vi "GeoData.vi"() -> ()   [LabVIEW 2017] (continued)
Currituck\tNC\tCurrituck County\tH1\n27927\t37053\tCorolla\tNC\tCurrituck County\tH1\n27917\t37053\tBarco\tNC\tCurrituck County\tH1\n27941\t37053\tHarbinger\tNC\tCurrituck County\tH1\n27916\t37053\tAydlett\tNC\tCurrituck County\tH1\n27966\t37053\tPowells point\tNC\tCurrituck County\tH1\n27939\t37053\tGrandy\tNC\tCurrituck County\tH1\n27958\t37053\tMoyock\tNC\tCurrituck County\tH1\n27949\t37055\tKitty hawk\tNC\tDare County\tH1\n27968\t37055\tRodanthe\tNC\tDare County\tH1\n27954\t37055\tManteo\tNC\tDare County\tH1\n27953\t37055\tManns harbor\tNC\tDare County\tH1\n27936\t37055\tFrisco\tNC\tDare County\tH1\n27959\t37055\tNags head\tNC\tDare County\tH1\n27981\t37055\tWanchese\tNC\tDare County\tH1\n27948\t37055\tKill devil hills\tNC\tDare County\tH1\n27943\t37055\tHatteras\tNC\tDare County\tH1\n27915\t37055\tAvon\tNC\tDare County\tH1\n27978\t37055\tStumpy point\tNC\tDare County\tH1\n27920\t37055\tBuxton\tNC\tDare County\tH1\n27360\t37057\tThomasville\tNC\tDavidson County\tH1\n27012\t37057\tClemmons\tNC\tDavidson County\tH1\n27374\t37057\tWelcome\tNC\tDavidson County\tH1\n27284\t37057\tKernersville\tNC\tDavidson County\tH1\n27262\t37057\tHigh point\tNC\tDavidson County\tH1\n28127\t37057\tNew london\tNC\tDavidson County\tH1\n27107\t37057\tWinston salem\tNC\tDavidson County\tH1\n27351\t37057\tSouthmont\tNC\tDavidson County\tH1\n27239\t37057\tDenton\tNC\tDavidson County\tH1\n27294\t37057\tLexington\tNC\tDavidson County\tH1\n27373\t37057\tWallburg\tNC\tDavidson County\tH1\n27299\t37057\tLinwood\tNC\tDavidson County\tH1\n27127\t37057\tWinston salem\tNC\tDavidson County\tH1\n27265\t37057\tHigh point\tNC\tDavidson County\tH1\n27292\t37057\tLexington\tNC\tDavidson County\tH1\n27295\t37057\tLexington\tNC\tDavidson County\tH1\n27293\t37057\tLexington\tNC\tDavidson County\tH1\n27014\t37059\tCooleemee\tNC\tDavie County\tH1\n28634\t37059\tHarmony\tNC\tDavie County\tH1\n27028\t37059\tMocksville\tNC\tDavie County\tH1\n27006\t37059\tAdvance\tNC\tDavie County\tH1\n28625\t37059\tStatesville\tNC\tDavie County\tH1\n27055\t37059\tYadkinville\tNC\tDavie County\tH1\n28458\t37061\tRose hill\tNC\tDuplin County\tH1\n28393\t37061\tTurkey\tNC\tDuplin County\tH1\n28365\t37061\tMount olive\tNC\tDuplin County\tH1\n28444\t37061\tHarrells\tNC\tDuplin County\tH1\n28572\t37061\tPink hill\tNC\tDuplin County\tH1\n28325\t37061\tCalypso\tNC\tDuplin County\tH1\n28508\t37061\tAlbertson\tNC\tDuplin County\tH1\n28341\t37061\tFaison\tNC\tDuplin County\tH1\n28453\t37061\tMagnolia\tNC\tDuplin County\tH1\n28525\t37061\tDeep run\tNC\tDuplin County\tH1\n28521\t37061\tChinquapin\tNC\tDuplin County\tH1\n28578\t37061\tSeven springs\tNC\tDuplin County\tH1\n28349\t37061\tKenansville\tNC\tDuplin County\tH1\n28398\t37061\tWarsaw\tNC\tDuplin County\tH1\n28464\t37061\tTeachey\tNC\tDuplin County\tH1\n28574\t37061\tRichlands\tNC\tDuplin County\tH1\n28478\t37061\tWillard\tNC\tDuplin County\tH1\n28518\t37061\tBeulaville\tNC\tDuplin County\tH1\n28466\t37061\tWallace\tNC\tDuplin County\tH1\n27704\t37063\tDurham\tNC\tDurham County\tH1\n27278\t37063\tHillsborough\tNC\tDurham County\tH1\n27503\t37063\tBahama\tNC\tDurham County\tH1\n27701\t37063\tDurham\tNC\tDurham County\tH1\n27709\t37063\tDurham\tNC\tDurham County\tH1\n27717\t37063\tDurham\tNC\tDurham County\tH1\n27712\t37063\tDurham\tNC\tDurham County\tH1\n27707\t37063\tDurham\tNC\tDurham County\tH1\n27713\t37063\tDurham\tNC\tDurham County\tH1\n27706\t37063\tDurham\tNC\tDurham County\tH1\n27560\t37063\tMorrisville\tNC\tDurham County\tH1\n27702\t37063\tDurham\tNC\tDurham County\tH1\n27715\t37063\tDurham\tNC\tDurham County\tH1\n27722\t37063\tDurham\tNC\tDurham County\tH1\n27708\t37063\tDurham\tNC\tDurham County\tH1\n27517\t37063\tChapel hill\tNC\tDurham County\tH1\n27583\t37063\tTimberlake\tNC\tDurham County\tH1\n27613\t37063\tRaleigh\tNC\tDurham County\tH1\n27705\t37063\tDurham\tNC\tDurham County\tH1\n27617\t37063\tRaleigh\tNC\tDurham County\tH1\n27703\t37063\tDurham\tNC\tDurham County\tH1\n27572\t37063\tRougemont\tNC\tDurham County\tH1\n27710\t37063\tDurham\tNC\tDurham County\tH1\n27809\t37065\tBattleboro\tNC\tEdgecombe County\tH1\n27886\t37065\tTarboro\tNC\tEdgecombe County\tH1\n27803\t37065\tRocky mount\tNC\tEdgecombe County\tH1\n27852\t37065\tMacclesfield\tNC\tEdgecombe County\tH1\n27843\t37065\tHobgood\tNC\tEdgecombe County\tH1\n27801\t37065\tRocky mount\tNC\tEdgecombe County\tH1\n27822\t37065\tElm city\tNC\tEdgecombe County\tH1\n27829\t37065\tFountain\tNC\tEdgecombe County\tH1\n27804\t37065\tRocky mount\tNC\tEdgecombe County\tH1\n27891\t37065\tWhitakers\tNC\tEdgecombe County\tH1\n27881\t37065\tSpeed\tNC\tEdgecombe County\tH1\n27819\t37065\tConetoe\tNC\tEdgecombe County\tH1\n27812\t37065\tBethel\tNC\tEdgecombe County\tH1\n27864\t37065\tPinetops\tNC\tEdgecombe County\tH1\n27802\t37065\tRocky mount\tNC\tEdgecombe County\tH1\n27815\t37065\tRocky mount\tNC\tEdgecombe County\tH1\n27834\t37065\tGreenville\tNC\tEdgecombe County\tH1\n27009\t37067\tBelews creek\tNC\tForsyth County\tH1\n27104\t37067\tWinston salem\tNC\tForsyth County\tH1\n27111\t37067\tWinston salem\tNC\tForsyth County\tH1\n27157\t37067\tWinston salem\tNC\tForsyth County\tH1\n27012\t37067\tClemmons\tNC\tForsyth County\tH1\n27021\t37067\tKing\tNC\tForsyth County\tH1\n27043\t37067\tPinnacle\tNC\tForsyth County\tH1\n27106\t37067\tWinston salem\tNC\tForsyth County\tH1\n27199\t37067\tWinston salem\tNC\tForsyth County\tH1\n27045\t37067\tRural hall\tNC\tForsyth County\tH1\n27101\t37067\tWinston salem\tNC\tForsyth County\tH1\n27115\t37067\tWinston salem\tNC\tForsyth County\tH1\n27284\t37067\tKernersville\tNC\tForsyth County\tH1\n27010\t37067\tBethania\tNC\tForsyth County\tH1\n27110\t37067\tWinston salem\tNC\tForsyth County\tH1\n27099\t37067\tRural hall\tNC\tForsyth County\tH1\n27019\t37067\tGermanton\tNC\tForsyth County\tH1\n27052\t37067\tWalnut cove\tNC\tForsyth County\tH1\n27357\t37067\tStokesdale\tNC\tForsyth County\tH1\n27117\t37067\tWinston salem\tNC\tForsyth County\tH1\n27094\t37067\tRural hall\tNC\tForsyth County\tH1\n27150\t37067\tWinston salem\tNC\tForsyth County\tH1\n27108\t37067\tWinston salem\tNC\tForsyth County\tH1\n27107\t37067\tWinston salem\tNC\tForsyth County\tH1\n27235\t37067\tColfax\tNC\tForsyth County\tH1\n27116\t37067\tWinston salem\tNC\tForsyth County\tH1\n27120\t37067\tWinston salem\tNC\tForsyth County\tH1\n27040\t37067\tPfafftown\tNC\tForsyth County\tH1\n27103\t37067\tWinston salem\tNC\tForsyth County\tH1\n27051\t37067\tWalkertown\tNC\tForsyth County\tH1\n27109\t37067\tWinston salem\tNC\tForsyth County\tH1\n27050\t37067\tTobaccoville\tNC\tForsyth County\tH1\n27285\t37067\tKernersville\tNC\tForsyth County\tH1\n27102\t37067\tWinston salem\tNC\tForsyth County\tH1\n27155\t37067\tWinston salem\tNC\tForsyth County\tH1\n27105\t37067\tWinston salem\tNC\tForsyth County\tH1\n27127\t37067\tWinston salem\tNC\tForsyth County\tH1\n27113\t37067\tWinston salem\tNC\tForsyth County\tH1\n27265\t37067\tHigh point\tNC\tForsyth County\tH1\n27023\t37067\tLewisville\tNC\tForsyth County\tH1\n27130\t37067\tWinston salem\tNC\tForsyth County\tH1\n27114\t37067\tWinston salem\tNC\tForsyth County\tH1\n27152\t37067\tWinston salem\tNC\tForsyth County\tH1\n27525\t37069\tFranklinton\tNC\tFranklin County\tH1\n27537\t37069\tHenderson\tNC\tFranklin County\tH1\n27587\t37069\tWake forest\tNC\tFranklin County\tH1\n27508\t37069\tBunn\tNC\tFranklin County\tH1\n27549\t37069\tLouisburg\tNC\tFranklin County\tH1\n27596\t37069\tYoungsville\tNC\tFranklin County\tH1\n27589\t37069\tWarrenton\tNC\tFranklin County\tH1\n27816\t37069\tCastalia\tNC\tFranklin County\tH1\n27544\t37069\tKittrell\tNC\tFranklin County\tH1\n27557\t37069\tMiddlesex\tNC\tFranklin County\tH1\n27597\t37069\tZebulon\tNC\tFranklin County\tH1\n27882\t37069\tSpring hope\tNC\tFranklin County\tH1\n28092\t37071\tLincolnton\tNC\tGaston County\tH1\n28077\t37071\tHigh shoals\tNC\tGaston County\tH1\n28052\t37071\tGastonia\tNC\tGaston County\tH1\n28006\t37071\tAlexis\tNC\tGaston County\tH1\n28101\t37071\tMc adenville\tNC\tGaston County\tH1\n28016\t37071\tBessemer city\tNC\tGaston County\tH1\n28032\t37071\tCramerton\tNC\tGaston County\tH1\n28054\t37071\tGastonia\tNC\tGaston County\tH1\n28080\t37071\tIron station\tNC\tGaston County\tH1\n28098\t37071\tLowell\tNC\tGaston County\tH1\n28034\t37071\tDallas\tNC\tGaston County\tH1\n28055\t37071\tGastonia\tNC\tGaston County\tH1\n28164\t37071\tStanley\tNC\tGaston County\tH1\n28012\t37071\tBelmont\tNC\tGaston County\tH1\n28120\t37071\tMount holly\tNC\tGaston County\tH1\n28021\t37071\tCherryville\tNC\tGaston County\tH1\n28056\t37071\tGastonia\tNC\tGaston County\tH1\n28033\t37071\tCrouse\tNC\tGaston County\tH1\n28053\t37071\tGastonia\tNC\tGaston County\tH1\n28086\t37071\tKings mountain\tNC\tGaston County\tH1\n27938\t37073\tGatesville\tNC\tGates County\tH1\n27969\t37073\tRoduco\tNC\tGates County\tH1\n27946\t37073\tHobbsville\tNC\tGates County\tH1\n27919\t37073\tBelvidere\tNC\tGates County\tH1\n27926\t37073\tCorapeake\tNC\tGates County\tH1\n27937\t37073\tGates\tNC\tGates County\tH1\n27979\t37073\tSunbury\tNC\tGates County\tH1\n27935\t37073\tEure\tNC\tGates County\tH1\n28702\t37075\tAlmond\tNC\tGraham County\tH1\n28733\t37075\tFontana dam\tNC\tGraham County\tH1\n28771\t37075\tRobbinsville\tNC\tGraham County\tH1\n27525\t37077\tFranklinton\tNC\tGranville County\tH1\n27587\t37077\tWake forest\tNC\tGranville County\tH1\n27582\t37077\tStovall\tNC\tGranville County\tH1\n27565\t37077\tOxford\tNC\tGranville County\tH1\n27596\t37077\tYoungsville\tNC\tGranville County\tH1\n27507\t37077\tBullock\tNC\tGranville County\tH1\n27574\t37077\tRoxboro\tNC\tGranville County\tH1\n27522\t37077\tCreedmoor\tNC\tGranville County\tH1\n27581\t37077\tStem\tNC\tGranville County\tH1\n27509\t37077\tButner\tNC\tGranville County\tH1\n27544\t37077\tKittrell\tNC\tGranville County\tH1\n27572\t37077\tRougemont\tNC\tGranville County\tH1\n28530\t37079\tGrifton\tNC\tGreene County\tH1\n28538\t37079\tHookerton\tNC\tGreene County\tH1\n27863\t37079\tPikeville\tNC\tGreene County\tH1\n28501\t37079\tKinston\tNC\tGreene County\tH1\n28554\t37079\tMaury\tNC\tGreene County\tH1\n27888\t37079\tWalstonburg\tNC\tGreene County\tH1\n27828\t37079\tFarmville\tNC\tGreene County\tH1\n27534\t37079\tGoldsboro\tNC\tGreene County\tH1\n28513\t37079\tAyden\tNC\tGreene County\tH1\n27883\t37079\tStantonsburg\tNC\tGreene County\tH1\n28551\t37079\tLa grange\tNC\tGreene County\tH1\n28580\t37079\tSnow hill\tNC\tGreene County\tH1\n27407\t37081\tGreensboro\tNC\tGuilford County\tH1\n27435\t37081\tGreensboro\tNC\tGuilford County\tH1\n27415\t37081\tGreensboro\tNC\tGuilford County\tH1\n27317\t37081\tRandleman\tNC\tGuilford County\tH1\n27310\t37081\tOak ridge\tNC\tGuilford County\tH1\n27403\t37081\tGreensboro\tNC\tGuilford County\tH1\n27408\t37081\tGreensboro\tNC\tGuilford County\tH1\n27455\t37081\tGreensboro\tNC\tGuilford County\tH1\n27425\t37081\tGreensboro\tNC\tGuilford County\tH1\n27417\t37081\tGreensboro\tNC\tGuilford County\tH1\n27268\t37081\tHigh point\tNC\tGuilford County\tH1\n27499\t37081\tGreensboro\tNC\tGuilford County\tH1\n27284\t37081\tKernersville\tNC\tGuilford County\tH1\n27320\t37081\tReidsville\tNC\tGuilford County\tH1\n27262\t37081\tHigh point\tNC\tGuilford County\tH1\n27313\t37081\tPleasant garden\tNC\tGuilford County\tH1\n27357\t37081\tStokesdale\tNC\tGuilford County\tH1\n27358\t37081\tSummerfield\tNC\tGuilford County\tH1\n27377\t37081\tWhitsett\tNC\tGuilford County\tH1\n27410\t37081\tGreensboro\tNC\tGuilford County\tH1\n27420\t37081\tGreensboro\tNC\tGuilford County\tH1\n27413\t37081\tGreensboro\tNC\tGuilford County\tH1\n27214\t37081\tBrowns summit\tNC\tGuilford County\tH1\n27235\t37081\tColfax\tNC\tGuilford County\tH1\n27260\t37081\tHigh point\tNC\tGuilford County\tH1\n27282\t37081\tJamestown\tNC\tGuilford County\tH1\n27261\t37081\tHigh point\tNC\tGuilford County\tH1\n27406\t37081\tGreensboro\tNC\tGuilford County\tH1\n27401\t37081\tGreensboro\tNC\tGuilford County\tH1\n27438\t37081\tGreensboro\tNC\tGuilford County\tH1\n27498\t37081\tGreensboro\tNC\tGuilford County\tH1\n27233\t37081\tClimax\tNC\tGuilford County\tH1\n27263\t37081\tHigh point\tNC\tGuilford County\tH1\n27409\t37081\tGreensboro\tNC\tGuilford County\tH1\n27416\t37081\tGreensboro\tNC\tGuilford County\tH1\n27404\t37081\tGreensboro\tNC\tGuilford County\tH1\n27244\t37081\tElon\tNC\tGuilford County\tH1\n27301\t37081\tMc leansville\tNC\tGuilford County\tH1\n27298\t37081\tLiberty\tNC\tGuilford County\tH1\n27429\t37081\tGreensboro\tNC\tGuilford County\tH1\n27419\t37081\tGreensboro\tNC\tGuilford County\tH1\n27412\t37081\tGreensboro\tNC\tGuilford County\tH1\n27411\t37081\tGreensboro\tNC\tGuilford County\tH1\n27342\t37081\tSedalia\tNC\tGuilford County\tH1\n27497\t37081\tGreensboro\tNC\tGuilford County\tH1\n27215\t37081\tBurlington\tNC\tGuilford County\tH1\n27249\t37081\tGibsonville\tNC\tGuilford County\tH1\n27265\t37081\tHigh point\tNC\tGuilford County\tH1\n27283\t37081\tJulian\tNC\tGuilford County\tH1\n27405\t37081\tGreensboro\tNC\tGuilford County\tH1\n27402\t37081\tGreensboro\tNC\tGuilford County\tH1\n27495\t37081\tGreensboro\tNC\tGuilford County\tH1\n27886\t37083\tTarboro\tNC\tHalifax County\tH1\n27850\t37083\tLittleton\tNC\tHalifax County\tH1\n27843\t37083\tHobgood\tNC\tHalifax County\tH1\n27870\t37083\tRoanoke rapids\tNC\tHalifax County\tH1\n27844\t37083\tHollister\tNC\tHalifax County\tH1\n27890\t37083\tWeldon\tNC\tHalifax County\tH1\n27823\t37083\tEnfield\tNC\tHalifax County\tH1\n27887\t37083\tTillery\tNC\tHalifax County\tH1\n27839\t37083\tHalifax\tNC\tHalifax County\tH1\n27874\t37083\tScotland neck\tNC\tHalifax County\tH1\n27891\t37083\tWhitakers\tNC\tHalifax County\tH1\n28326\t37085\tCameron\tNC\tHarnett County\tH1\n28334\t37085\tDunn\tNC\tHarnett County\tH1\n27330\t37085\tSanford\tNC\tHarnett County\tH1\n27504\t37085\tBenson\tNC\tHarnett County\tH1\n27526\t37085\tFuquay varina\tNC\tHarnett County\tH1\n28368\t37085\tOlivia\tNC\tHarnett County\tH1\n27501\t37085\tAngier\tNC\tHarnett County\tH1\n27592\t37085\tWillow spring\tNC\tHarnett County\tH1\n28323\t37085\tBunnlevel\tNC\tHarnett County\tH1\n27332\t37085\tSanford\tNC\tHarnett County\tH1\n27521\t37085\tCoats\tNC\tHarnett County\tH1\n28356\t37085\tLinden\tNC\tHarnett County\tH1\n28390\t37085\tSpring lake\tNC\tHarnett County\tH1\n27506\t37085\tBuies creek\tNC\tHarnett County\tH1\n27543\t37085\tKipling\tNC\tHarnett County\tH1\n28339\t37085\tErwin\tNC\tHarnett County\tH1\n27505\t37085\tBroadway\tNC\tHarnett County\tH1\n27540\t37085\tHolly springs\tNC\tHarnett County\tH1\n27546\t37085\tLillington\tNC\tHarnett County\tH1\n27552\t37085\tMamers\tNC\tHarnett County\tH1\n28715\t37087\tCandler\tNC\tHaywood County\tH1\n28719\t37087\tCherokee\tNC\tHaywood County\tH1\n28723\t37087\tCullowhee\tNC\tHaywood County\tH1\n28738\t37087\tHazelwood\tNC\tHaywood County\tH1\n28721\t37087\tClyde\tNC\tHaywood County\tH1\n28779\t37087\tSylva\tNC\tHaywood County\tH1\n28785\t37087\tWaynesville\tNC\tHaywood County\tH1\n28745\t37087\tLake junaluska\tNC\tHaywood County\tH1\n28743\t37087\tHot springs\tNC\tHaywood County\tH1\n28716\t37087\tCanton\tNC\tHaywood County\tH1\n28751\t37087\tMaggie valley\tNC\tHaywood County\tH1\n28786\t37087\tWaynesville\tNC\tHaywood County\tH1\n28766\t37089\tPenrose\tNC\tHenderson County\tH1\n28724\t37089\tDana\tNC\tHenderson County\tH1\n28735\t37089\tGerton\tNC\tHenderson County\tH1\n28793\t37089\tHendersonville\tNC\tHenderson County\tH1\n28739\t37089\tHendersonville\tNC\tHenderson County\tH1\n28742\t37089\tHorse shoe\tNC\tHenderson County\tH1\n28784\t37089\tTuxedo\tNC\tHenderson County\tH1\n28758\t37089\tMountain home\tNC\tHenderson County\tH1\n28732\t37089\tFletcher\tNC\tHenderson County\tH1\n28756\t37089\tMill spring\tNC\tHenderson County\tH1\n28731\t37089\tFlat rock\tNC\tHenderson County\tH1\n28790\t37089\tZirconia\tNC\tHenderson County\tH1\n28729\t37089\tEtowah\tNC\tHenderson County\tH1\n28704\t37089\tArden\tNC\tHenderson County\tH1\n28768\t37089\tPisgah forest\tNC\tHenderson County\tH1\n28727\t37089\tEdneyville\tNC\tHenderson County\tH1\n28711\t37089\tBlack mountain\tNC\tHenderson County\tH1\n28710\t37089\tBat cave\tNC\tHenderson County\tH1\n28726\t37089\tEast flat rock\tNC\tHenderson County\tH1\n28760\t37089\tNaples\tNC\tHenderson County\tH1\n28773\t37089\tSaluda\tNC\tHenderson County\tH1\n28791\t37089\tHendersonville\tNC\tHenderson County\tH1\n28759\t37089\tMills river\tNC\tHenderson County\tH1\n28792\t37089\tHendersonville\tNC\tHenderson County\tH1\n27897\t37091\tWoodland\tNC\tHertford County\tH1\n27942\t37091\tHarrellsville\tNC\tHertford County\tH1\n27805\t37091\tAulander\tNC\tHertford County\tH1\n27855\t37091\tMurfreesboro\tNC\tHertford County\tH1\n27910\t37091\tAhoskie\tNC\tHertford County\tH1\n27922\t37091\tCofield\tNC\tHertford County\tH1\n27986\t37091\tWinton\tNC\tHertford County\tH1\n27818\t37091\tComo\tNC\tHertford County\tH1\n28371\t37093\tParkton\tNC\tHoke County\tH1\n28306\t37093\tFayetteville\tNC\tHoke County\tH1\n28315\t37093\tAberdeen\tNC\tHoke County\tH1\n28364\t37093\tMaxton\tNC\tHoke County\tH1\n28304\t37093\tFayetteville\tNC\tHoke County\tH1\n28377\t37093\tRed springs\tNC\tHoke County\tH1\n28386\t37093\tShannon\tNC\tHoke County\tH1\n28376\t37093\tRaeford\tNC\tHoke County\tH1\n28357\t37093\tLumber bridge\tNC\tHoke County\tH1\n27860\t37095\tPantego\tNC\tHyde County\tH1\n27810\t37095\tBelhaven\tNC\tHyde County\tH1\n27875\t37095\tScranton\tNC\tHyde County\tH1\n27826\t37095\tFairfield\tNC\tHyde County\tH1\n27824\t37095\tEngelhard\tNC\tHyde County\tH1\n27960\t37095\tOcracoke\tNC\tHyde County\tH1\n27885\t37095\tSwanquarter\tNC\tHyde County\tH1\n28677\t37097\tStatesville\tNC\tIredell County\tH1\n28166\t37097\tTroutman\tNC\tIredell County\tH1\n28636\t37097\tHiddenite\tNC\tIredell County\tH1\n28634\t37097\tHarmony\tNC\tIredell County\tH1\n28123\t37097\tMount mourne\tNC\tIredell County\tH1\n28699\t37097\tScotts\tNC\tIredell County\tH1\n27028\t37097\tMocksville\tNC\tIredell County\tH1\n28688\t37097\tTurnersburg\tNC\tIredell County\tH1\n28660\t37097\tOlin\tNC\tIredell County\tH1\n28117\t37097\tMooresville\tNC\tIredell County\tH1\n28125\t37097\tMount ulla\tNC\tIredell County\tH1\n28687\t37097\tStatesville\tNC\tIredell County\tH1\n28010\t37097\tBarium springs\tNC\tIredell County\tH1\n28625\t37097\tStatesville\tNC\tIredell County\tH1\n28036\t37097\tDavidson\tNC\tIredell County\tH1\n27013\t37097\tCleveland\tNC\tIredell County\tH1\n27020\t37097\tHamptonville\tNC\tIredell County\tH1\n27055\t37097\tYadkinville\tNC\tIredell County\tH1\n28678\t37097\tStony point\tNC\tIredell County\tH1\n28115\t37097\tMooresville\tNC\tIredell County\tH1\n28689\t37097\tUnion grove\tNC\tIredell County\tH1\n28719\t37099\tCherokee\tNC\tJackson County\tH1\n28723\t37099\tCullowhee\tNC\tJackson County\tH1\n28747\t37099\tLake toxaway\tNC\tJackson County\tH1\n28707\t37099\tBalsam\tNC\tJackson County\tH1\n28741\t37099\tHighlands\tNC\tJackson County\tH1\n28779\t37099\tSylva\tNC\tJackson County\tH1\n28788\t37099\tWebster\tNC\tJackson County\tH1\n28717\t37099\tCashiers\tNC\tJackson County\tH1\n28789\t37099\tWhittier\tNC\tJackson County\tH1\n28783\t37099\tTuckasegee\tNC\tJackson County\tH1\n28774\t37099\tSapphire\tNC\tJackson County\tH1\n28725\t37099\tDillsboro\tNC\tJackson County\tH1\n28736\t37099\tGlenville\tNC\tJackson County\tH1\n28751\t37099\tMaggie valley\tNC\tJackson County\tH1\n27542\t37101\tKenly\tNC\tJohnston County\tH1\n27610\t37101\tRaleigh\tNC\tJohnston County\tH1\n28334\t37101\tDunn\tNC\tJohnston County\tH1\n27504\t37101\tBenson\tNC\tJohnston County\tH1\n27524\t37101\tFour oaks\tNC\tJohnston County\tH1\n27863\t37101\tPikeville\tNC\tJohnston County\tH1\n27501\t37101\tAngier\tNC\tJohnston County\tH1\n27569\t37101\tPrinceton\tNC\tJohnston County\tH1\n27520\t37101\tClayton\tNC\tJohnston County\tH1\n27592\t37101\tWillow spring\tNC\tJohnston County\tH1\n28366\t37101\tNewton grove\tNC\tJohnston County\tH1\n27529\t37101\tGarner\tNC\tJohnston County\tH1\n27568\t37101\tPine level\tNC\tJohnston County\tH1\n27593\t37101\tWilsons mills\tNC\tJohnston County\tH1\n27591\t37101\tWendell\tNC\tJohnston County\tH1\n27577\t37101\tSmithfield\tNC\tJohnston County\tH1\n27603\t37101\tRaleigh\tNC\tJohnston County\tH1\n27555\t37101\tMicro\tNC\tJohnston County\tH1\n27527\t37101\tClayton\tNC\tJohnston County\tH1\n27557\t37101\tMiddlesex\tNC\tJohnston County\tH1\n27576\t37101\tSelma\tNC\tJohnston County\tH1\n27597\t37101\tZebulon\tNC\tJohnston County\tH1\n27528\t37101\tClayton\tNC\tJohnston County\tH1\n28501\t37103\tKinston\tNC\tJones County\tH1\n28522\t37103\tComfort\tNC\tJones County\tH1\n28572\t37103\tPink hill\tNC\tJones County\tH1\n28573\t37103\tPollocksville\tNC\tJones County\tH1\n28526\t37103\tDover\tNC\tJones County\tH1\n28555\t37103\tMaysville\tNC\tJones County\tH1\n28504\t37103\tKinston\tNC\tJones County\tH1\n28585\t37103\tTrenton\tNC\tJones County\tH1\n28574\t37103\tRichlands\tNC\tJones County\tH1\n28562\t37103\tNew bern\tNC\tJones County\tH1\n28326\t37105\tCameron\tNC\tLee County\tH1\n27207\t37105\tBear creek\tNC\tLee County\tH1\n27330\t37105\tSanford\tNC\tLee County\tH1\n27331\t37105\tSanford\tNC\tLee County\tH1\n28355\t37105\tLemon springs\tNC\tLee County\tH1\n27332\t37105\tSanford\tNC\tLee County\tH1\n27505\t37105\tBroadway\tNC\tLee County\tH1\n28530\t37107\tGrifton\tNC\tLenoir County\tH1\n28538\t37107\tHookerton\tNC\tLenoir County\tH1\n28501\t37107\tKinston\tNC\tLenoir County\tH1\n28572\t37107\tPink hill\tNC\tLenoir County\tH1\n28526\t37107\tDover\tNC\tLenoir County\tH1\n28525\t37107\tDeep run\tNC\tLenoir County\tH1\n28578\t37107\tSeven springs\tNC\tLenoir County\tH1\n28504\t37107\tKinston\tNC\tLenoir County\tH1\n28551\t37107\tLa grange\tNC\tLenoir County\tH1\n28580\t37107\tSnow hill\tNC\tLenoir County\tH1\n28092\t37109\tLincolnton\tNC\tLincoln County\tH1\n28006\t37109\tAlexis\tNC\tLincoln County\tH1\n28650\t37109\tMaiden\tNC\tLincoln County\tH1\n28016\t37109\tBessemer city\tNC\tLincoln County\tH1\n28080\t37109\tIron station\tNC\tLincoln County\tH1\n28093\t37109\tLincolnton\tNC\tLincoln County\tH1\n28673\t37109\tSherrills ford\tNC\tLincoln County\tH1\n28034\t37109\tDallas\tNC\tLincoln County\tH1\n28037\t37109\tDenver\tNC\tLincoln County\tH1\n28164\t37109\tStanley\tNC\tLincoln County\tH1\n28021\t37109\tCherryville\tNC\tLincoln County\tH1\n28168\t37109\tVale\tNC\tLincoln County\tH1\n28033\t37109\tCrouse\tNC\tLincoln County\tH1\n28090\t37109\tLawndale\tNC\tLincoln County\tH1\n28167\t37111\tUnion mills\tNC\tMcDowell County\tH1\n28752\t37111\tMarion\tNC\tMcDowell County\tH1\n28655\t37111\tMorganton\tNC\tMcDowell County\tH1\n28714\t37111\tBurnsville\tNC\tMcDowell County\tH1\n28777\t37111\tSpruce pine\tNC\tMcDowell County\tH1\n28761\t37111\tNebo\tNC\tMcDowell County\tH1\n28762\t37111\tOld fort\tNC\tMcDowell County\tH1\n28711\t37111\tBlack mountain\tNC\tMcDowell County\tH1\n28657\t37111\tNewland\tNC\tMcDowell County\tH1\n28749\t37111\tLittle switzerland\tNC\tMcDowell County\tH1\n28713\t37113\tBryson city\tNC\tMacon County\tH1\n28734\t37113\tFranklin\tNC\tMacon County\tH1\n28741\t37113\tHighlands\tNC\tMacon County\tH1\n28779\t37113\tSylva\tNC\tMacon County\tH1\n28775\t37113\tScaly mountain\tNC\tMacon County\tH1\n28763\t37113\tOtto\tNC\tMacon County\tH1\n28781\t37113\tTopton\tNC\tMacon County\tH1\n28744\t37113\tFranklin\tNC\tMacon County\tH1\n28701\t37115\tAlexander\tNC\tMadison County\tH1\n28714\t37115\tBurnsville\tNC\tMadison County\tH1\n28743\t37115\tHot springs\tNC\tMadison County\tH1\n28787\t37115\tWeaverville\tNC\tMadison County\tH1\n28753\t37115\tMarshall\tNC\tMadison County\tH1\n28748\t37115\tLeicester\tNC\tMadison County\tH1\n28754\t37115\tMars hill\tNC\tMadison County\tH1\n27861\t37117\tParmele\tNC\tMartin County\tH1\n27843\t37117\tHobgood\tNC\tMartin County\tH1\n27962\t37117\tPlymouth\tNC\tMartin County\tH1\n27846\t37117\tJamesville\tNC\tMartin County\tH1\n27889\t37117\tWashington\tNC\tMartin County\tH1\n27840\t37117\tHamilton\tNC\tMartin County\tH1\n27825\t37117\tEveretts\tNC\tMartin County\tH1\n27857\t37117\tOak city\tNC\tMartin County\tH1\n27812\t37117\tBethel\tNC\tMartin County\tH1\n27892\t37117\tWilliamston\tNC\tMartin County\tH1\n27871\t37117\tRobersonville\tNC\tMartin County\tH1\n27841\t37117\tHassell\tNC\tMartin County\tH1\n28031\t37119\tCornelius\tNC\tMecklenburg County\tH1\n28106\t37119\tMatthews\tNC\tMecklenburg County\tH1\n28203\t37119\tCharlotte\tNC\tMecklenburg County\tH1\n28210\t37119\tCharlotte\tNC\tMecklenburg County\tH1\n28212\t37119\tCharlotte\tNC\tMecklenburg County\tH1\n28217\t37119\tCharlotte\tNC\tMecklenburg County\tH1\n28226\t37119\tCharlotte\tNC\tMecklenburg County\tH1\n28214\t37119\tCharlotte\tNC\tMecklenburg County\tH1\n28278\t37119\tCharlotte\tNC\tMecklenburg County\tH1\n28282\t37119\tCharlotte\tNC\tMecklenburg County\tH1\n28130\t37119\tPaw creek\tNC\tMecklenburg County\tH1\n28126\t37119\tNewell\tNC\tMecklenburg County\tH1\n28234\t37119\tCharlotte\tNC\tMecklenburg County\tH1\n28274\t37119\tCharlotte\tNC\tMecklenburg County\tH1\n28035\t37119\tDavidson\tNC\tMecklenburg County\tH1\n28223\t37119\tCharlotte\tNC\tMecklenburg County\tH1\n28206\t37119\tCharlotte\tNC\tMecklenburg County\tH1\n28269\t37119\tCharlotte\tNC\tMecklenburg County\tH1\n28271\t37119\tCharlotte\tNC\tMecklenburg County\tH1\n28221\t37119\tCharlotte\tNC\tMecklenburg County\tH1\n28247\t37119\tCharlotte\tNC\tMecklenburg County\tH1\n28224\t37119\tCharlotte\tNC\tMecklenburg County\tH1\n28284\t37119\tCharlotte\tNC\tMecklenburg County\tH1\n28233\t37119\tCharlotte\tNC\tMecklenburg County\tH1\n28134\t37119\tPineville\tNC\tMecklenburg County\tH1\n28202\t37119\tCharlotte\tNC\tMecklenburg County\tH1\n28209\t37119\tCharlotte\tNC\tMecklenburg County\tH1\n28229\t37119\tCharlotte\tNC\tMecklenburg County\tH1\n28266\t37119\tCharlotte\tNC\tMecklenburg County\tH1\n28222\t37119\tCharlotte\tNC\tMecklenburg County\tH1\n28244\t37119\tCharlotte\tNC\tMecklenburg County\tH1\n28285\t37119\tCharlotte\tNC\tMecklenburg County\tH1\n28235\t37119\tCharlotte\tNC\tMecklenburg County\tH1\n28281\t37119\tCharlotte\tNC\tMecklenburg County\tH1\n28208\t37119\tCharlotte\tNC\tMecklenburg County\tH1\n28207\t37119\tCharlotte\tNC\tMecklenburg County\tH1\n28213\t37119\tCharlotte\tNC\tMecklenburg County\tH1\n28256\t37119\tCharlotte\tNC\tMecklenburg County\tH1\n28227\t37119\tCharlotte\tNC\tMecklenburg County\tH1\n28273\t37119\tCharlotte\tNC\tMecklenburg County\tH1\n28232\t37119\tCharlotte\tNC\tMecklenburg County\tH1\n28219\t37119\tCharlotte\tNC\tMecklenburg County\tH1\n28231\t37119\tCharlotte\tNC\tMecklenburg County\tH1\n28105\t37119\tMatthews\tNC\tMecklenburg County\tH1\n28277\t37119\tCharlotte\tNC\tMecklenburg County\tH1\n28287\t37119\tCharlotte\tNC\tMecklenburg County\tH1\n28201\t37119\tCharlotte\tNC\tMecklenburg County\tH1\n28288\t37119\tCharlotte\tNC\tMecklenburg County\tH1\n28107\t37119\tMidland\tNC\tMecklenburg County\tH1\n28205\t37119\tCharlotte\tNC\tMecklenburg County\tH1\n28211\t37119\tCharlotte\tNC\tMecklenburg County\tH1\n28216\t37119\tCharlotte\tNC\tMecklenburg County\tH1\n28220\t37119\tCharlotte\tNC\tMecklenburg County\tH1\n28241\t37119\tCharlotte\tNC\tMecklenburg County\tH1\n28280\t37119\tCharlotte\tNC\tMecklenburg County\tH1\n28070\t37119\tHuntersville\tNC\tMecklenburg County\tH1\n28297\t37119\tCharlotte\tNC\tMecklenburg County\tH1\n28246\t37119\tCharlotte\tNC\tMecklenburg County\tH1\n28036\t37119\tDavidson\tNC\tMecklenburg County\tH1\n28079\t37119\tIndian trail\tNC\tMecklenburg County\tH1\n28204\t37119\tCharlotte\tNC\tMecklenburg County\tH1\n28215\t37119\tCharlotte\tNC\tMecklenburg County\tH1\n28270\t37119\tCharlotte\tNC\tMecklenburg County\tH1\n28299\t37119\tCharlotte\tNC\tMecklenburg County\tH1\n28230\t37119\tCharlotte\tNC\tMecklenburg County\tH1\n28236\t37119\tCharlotte\tNC\tMecklenburg County\tH1\n28228\t37119\tCharlotte\tNC\tMecklenburg County\tH1\n28078\t37119\tHuntersville\tNC\tMecklenburg County\tH1\n28104\t37119\tMatthews\tNC\tMecklenburg County\tH1\n28262\t37119\tCharlotte\tNC\tMecklenburg County\tH1\n28237\t37119\tCharlotte\tNC\tMecklenburg County\tH1\n28714\t37121\tBurnsville\tNC\tMitchell County\tH1\n28777\t37121\tSpruce pine\tNC\tMitchell County\tH1\n28765\t37121\tPenland\tNC\tMitchell County\tH1\n28740\t37121\tGreen mountain\tNC\tMitchell County\tH1\n28705\t37121\tBakersville\tNC\tMitchell County\tH1\n28338\t37123\tEllerbe\tNC\tMontgomery County\tH1\n27306\t37123\tMount gilead\tNC\tMontgomery County\tH1\n27371\t37123\tTroy\tNC\tMontgomery County\tH1\n27242\t37123\tEagle springs\tNC\tMontgomery County\tH1\n27341\t37123\tSeagrove\tNC\tMontgomery County\tH1\n27356\t37123\tStar\tNC\tMontgomery County\tH1\n28127\t37123\tNew london\tNC\tMontgomery County\tH1\n27229\t37123\tCandor\tNC\tMontgomery County\tH1\n27239\t37123\tDenton\tNC\tMontgomery County\tH1\n27209\t37123\tBiscoe\tNC\tMontgomery County\tH1\n27281\t37123\tJackson springs\tNC\tMontgomery County\tH1\n27247\t37123\tEther\tNC\tMontgomery County\tH1\n28326\t37125\tCameron\tNC\tMoore County\tH1\n27330\t37125\tSanford\tNC\tMoore County\tH1\n27376\t37125\tWest end\tNC\tMoore County\tH1\n28374\t37125\tPinehurst\tNC\tMoore County\tH1\n27325\t37125\tRobbins\tNC\tMoore County\tH1\n28347\t37125\tHoffman\tNC\tMoore County\tH1\n27242\t37125\tEagle springs\tNC\tMoore County\tH1\n27341\t37125\tSeagrove\tNC\tMoore County\tH1\n27356\t37125\tStar\tNC\tMoore County\tH1\n28315\t37125\tAberdeen\tNC\tMoore County\tH1\n28394\t37125\tVass\tNC\tMoore County\tH1\n28388\t37125\tSouthern pines\tNC\tMoore County\tH1\n28350\t37125\tLakeview\tNC\tMoore County\tH1\n27259\t37125\tHighfalls\tNC\tMoore County\tH1\n27252\t37125\tGoldston\tNC\tMoore County\tH1\n28373\t37125\tPinebluff\tNC\tMoore County\tH1\n27209\t37125\tBiscoe\tNC\tMoore County\tH1\n27208\t37125\tBennett\tNC\tMoore County\tH1\n28327\t37125\tCarthage\tNC\tMoore County\tH1\n28370\t37125\tPinehurst\tNC\tMoore County\tH1\n27281\t37125\tJackson springs\tNC\tMoore County\tH1\n28387\t37125\tSouthern pines\tNC\tMoore County\tH1\n27809\t37127\tBattleboro\tNC\tNash County\tH1\n27803\t37127\tRocky mount\tNC\tNash County\tH1\n27807\t37127\tBailey\tNC\tNash County\tH1\n27856\t37127\tNashville\tNC\tNash County\tH1\n27878\t37127\tSharpsburg\tNC\tNash County\tH1\n27822\t37127\tElm city\tNC\tNash County\tH1\n27880\t37127\tSims\tNC\tNash County\tH1\n27816\t37127\tCastalia\tNC\tNash County\tH1\n27804\t37127\tRocky mount\tNC\tNash County\tH1\n27896\t37127\tWilson\tNC\tNash County\tH1\n27891\t37127\tWhitakers\tNC\tNash County\tH1\n27868\t37127\tRed oak\tNC\tNash County\tH1\n27557\t37127\tMiddlesex\tNC\tNash County\tH1\n27597\t37127\tZebulon\tNC\tNash County\tH1\n27882\t37127\tSpring hope\tNC\tNash County\tH1\n28409\t37129\tWilmington\tNC\tNew Hanover County\tH1\n28429\t37129\tCastle hayne\tNC\tNew Hanover County\tH1\n28428\t37129\tCarolina beach\tNC\tNew Hanover County\tH1\n28404\t37129\tWilmington\tNC\tNew Hanover County\tH1\n28411\t37129\tWilmington\tNC\tNew Hanover County\tH1\n28449\t37129\tKure beach\tNC\tNew Hanover County\tH1\n28410\t37129\tWilmington\tNC\tNew Hanover County\tH1\n28403\t37129\tWilmington\tNC\tNew Hanover County\tH1\n28401\t37129\tWilmington\tNC\tNew Hanover County\tH1\n28480\t37129\tWrightsville beach\tNC\tNew Hanover County\tH1\n28408\t37129\tWilmington\tNC\tNew Hanover County\tH1\n28405\t37129\tWilmington\tNC\tNew Hanover County\tH1\n28406\t37129\tWilmington\tNC\tNew Hanover County\tH1\n28402\t37129\tWilmington\tNC\tNew Hanover County\tH1\n28412\t37129\tWilmington\tNC\tNew Hanover County\tH1\n27831\t37131\tGarysburg\tNC\tNorthampton County\tH1\n27862\t37131\tPendleton\tNC\tNorthampton County\tH1\n27897\t37131\tWoodland\tNC\tNorthampton County\tH1\n27866\t37131\tPleasant hill\tNC\tNorthampton County\tH1\n27853\t37131\tMargarettsville\tNC\tNorthampton County\tH1\n27876\t37131\tSeaboard\tNC\tNorthampton County\tH1\n27805\t37131\tAulander\tNC\tNorthampton County\tH1\n27855\t37131\tMurfreesboro\tNC\tNorthampton County\tH1\n27845\t37131\tJackson\tNC\tNorthampton County\tH1\n27832\t37131\tGaston\tNC\tNorthampton County\tH1\n27869\t37131\tRich square\tNC\tNorthampton County\tH1\n27877\t37131\tSevern\tNC\tNorthampton County\tH1\n27820\t37131\tConway\tNC\tNorthampton County\tH1\n27842\t37131\tHenrico\tNC\tNorthampton County\tH1\n27867\t37131\tPotecasi\tNC\tNorthampton County\tH1\n28541\t37133\tJacksonville\tNC\tOnslow County\tH1\n28445\t37133\tHolly ridge\tNC\tOnslow County\tH1\n28582\t37133\tStella\tNC\tOnslow County\tH1\n28547\t37133\tCamp lejeune\tNC\tOnslow County\tH1\n28584\t37133\tSwansboro\tNC\tOnslow County\tH1\n28555\t37133\tMaysville\tNC\tOnslow County\tH1\n28521\t37133\tChinquapin\tNC\tOnslow County\tH1\n28546\t37133\tJacksonville\tNC\tOnslow County\tH1\n28454\t37133\tMaple hill\tNC\tOnslow County\tH1\n28460\t37133\tSneads ferry\tNC\tOnslow County\tH1\n28540\t37133\tJacksonville\tNC\tOnslow County\tH1\n28543\t37133\tTarawa terrace\tNC\tOnslow County\tH1\n28539\t37133\tHubert\tNC\tOnslow County\tH1\n28574\t37133\tRichlands\tNC\tOnslow County\tH1\n28518\t37133\tBeulaville\tNC\tOnslow County\tH1\n28545\t37133\tMccutcheon field\tNC\tOnslow County\tH1\n28544\t37133\tMidway park\tNC\tOnslow County\tH1\n28542\t37133\tCamp lejeune\tNC\tOnslow County\tH1\n27278\t37135\tHillsborough\tNC\tOrange County\tH1\n27599\t37135\tChapel hill\tNC\tOrange County\tH1\n27514\t37135\tChapel hill\tNC\tOrange County\tH1\n27712\t37135\tDurham\tNC\tOrange County\tH1\n27707\t37135\tDurham\tNC\tOrange County\tH1\n27243\t37135\tEfland\tNC\tOrange County\tH1\n27312\t37135\tPittsboro\tNC\tOrange County\tH1\n27516\t37135\tChapel hill\tNC\tOrange County\tH1\n27231\t37135\tCedar grove\tNC\tOrange County\tH1\n27302\t37135\tMebane\tNC\tOrange County\tH1\n27510\t37135\tCarrboro\tNC\tOrange County\tH1\n27517\t37135\tChapel hill\tNC\tOrange County\tH1\n27583\t37135\tTimberlake\tNC\tOrange County\tH1\n27705\t37135\tDurham\tNC\tOrange County\tH1\n27314\t37135\tProspect hill\tNC\tOrange County\tH1\n27541\t37135\tHurdle mills\tNC\tOrange County\tH1\n27515\t37135\tChapel hill\tNC\tOrange County\tH1\n27572\t37135\tRougemont\tNC\tOrange County\tH1\n28560\t37137\tNew bern\tNC\tPamlico County\tH1\n28552\t37137\tLowland\tNC\tPamlico County\tH1\n28509\t37137\tAlliance\tNC\tPamlico County\tH1\n28571\t37137\tOriental\tNC\tPamlico County\tH1\n28515\t37137\tBayboro\tNC\tPamlico County\tH1\n28510\t37137\tArapahoe\tNC\tPamlico County\tH1\n28587\t37137\tVandemere\tNC\tPamlico County\tH1\n28583\t37137\tStonewall\tNC\tPamlico County\tH1\n28529\t37137\tGrantsboro\tNC\tPamlico County\tH1\n28556\t37137\tMerritt\tNC\tPamlico County\tH1\n28537\t37137\tHobucken\tNC\tPamlico County\tH1\n27906\t37139\tElizabeth city\tNC\tPasquotank County\tH1\n27907\t37139\tElizabeth city\tNC\tPasquotank County\tH1\n27909\t37139\tElizabeth city\tNC\tPasquotank County\tH1\n28445\t37141\tHolly ridge\tNC\tPender County\tH1\n28448\t37141\tKelly\tNC\tPender County\tH1\n28411\t37141\tWilmington\tNC\tPender County\tH1\n28435\t37141\tCurrie\tNC\tPender County\tH1\n28401\t37141\tWilmington\tNC\tPender County\tH1\n28454\t37141\tMaple hill\tNC\tPender County\tH1\n28447\t37141\tIvanhoe\tNC\tPender County\tH1\n28425\t37141\tBurgaw\tNC\tPender County\tH1\n28457\t37141\tRocky point\tNC\tPender County\tH1\n28478\t37141\tWillard\tNC\tPender County\tH1\n28421\t37141\tAtkinson\tNC\tPender County\tH1\n28443\t37141\tHampstead\tNC\tPender County\tH1\n28466\t37141\tWallace\tNC\tPender County\tH1\n27985\t37143\tWinfall\tNC\tPerquimans County\tH1\n27944\t37143\tHertford\tNC\tPerquimans County\tH1\n27946\t37143\tHobbsville\tNC\tPerquimans County\tH1\n27919\t37143\tBelvidere\tNC\tPerquimans County\tH1\n27980\t37143\tTyner\tNC\tPerquimans County\tH1\n27932\t37143\tEdenton\tNC\tPerquimans County\tH1\n27343\t37145\tSemora\tNC\tPerson County\tH1\n27573\t37145\tRoxboro\tNC\tPerson County\tH1\n27565\t37145\tOxford\tNC\tPerson County\tH1\n27574\t37145\tRoxboro\tNC\tPerson County\tH1\n27231\t37145\tCedar grove\tNC\tPerson County\tH1\n27583\t37145\tTimberlake\tNC\tPerson County\tH1\n27541\t37145\tHurdle mills\tNC\tPerson County\tH1\n27305\t37145\tMilton\tNC\tPerson County\tH1\n27291\t37145\tLeasburg\tNC\tPerson County\tH1\n27572\t37145\tRougemont\tNC\tPerson County\tH1\n27886\t37147\tTarboro\tNC\tPitt County\tH1\n28530\t37147\tGrifton\tNC\tPitt County\tH1\n27852\t37147\tMacclesfield\tNC\tPitt County\tH1\n27827\t37147\tFalkland\tNC\tPitt County\tH1\n27858\t37147\tGreenville\tNC\tPitt County\tH1\n28590\t37147\tWinterville\tNC\tPitt County\tH1\n28586\t37147\tVanceboro\tNC\tPitt County\tH1\n27829\t37147\tFountain\tNC\tPitt County\tH1\n27837\t37147\tGrimesland\tNC\tPitt County\tH1\n27889\t37147\tWashington\tNC\tPitt County\tH1\n27888\t37147\tWalstonburg\tNC\tPitt County\tH1\n27817\t37147\tChocowinity\tNC\tPitt County\tH1\n27828\t37147\tFarmville\tNC\tPitt County\tH1\n27835\t37147\tGreenville\tNC\tPitt County\tH1\n27836\t37147\tGreenville\tNC\tPitt County\tH1\n27879\t37147\tSimpson\tNC\tPitt County\tH1\n27811\t37147\tBellarthur\tNC\tPitt County\tH1\n27812\t37147\tBethel\tNC\tPitt County\tH1\n28513\t37147\tAyden\tNC\tPitt County\tH1\n27834\t37147\tGreenville\tNC\tPitt County\tH1\n27871\t37147\tRobersonville\tNC\tPitt County\tH1\n27884\t37147\tStokes\tNC\tPitt County\tH1\n27833\t37147\tGreenville\tNC\tPitt County\tH1\n28139\t37149\tRutherfordton\tNC\tPolk County\tH1\n28722\t37149\tColumbus\tNC\tPolk County\tH1\n28756\t37149\tMill spring\tNC\tPolk County\tH1\n28782\t37149\tTryon\tNC\tPolk County\tH1\n28731\t37149\tFlat rock\tNC\tPolk County\tH1\n28746\t37149\tLake lure\tNC\tPolk County\tH1\n28750\t37149\tLynn\tNC\tPolk County\tH1\n28773\t37149\tSaluda\tNC\tPolk County\tH1\n28792\t37149\tHendersonville\tNC\tPolk County\tH1\n27360\t37151\tThomasville\tNC\tRandolph County\tH1\n27230\t37151\tCedar falls\tNC\tRandolph County\tH1\n27203\t37151\tAsheboro\tNC\tRandolph County\tH1\n27317\t37151\tRandleman\tNC\tRandolph County\tH1\n27344\t37151\tSiler city\tNC\tRandolph County\tH1\n27371\t37151\tTroy\tNC\tRandolph County\tH1\n27205\t37151\tAsheboro\tNC\tRandolph County\tH1\n27325\t37151\tRobbins\tNC\tRandolph County\tH1\n27262\t37151\tHigh point\tNC\tRandolph County\tH1\n27313\t37151\tPleasant garden\tNC\tRandolph County\tH1\n27341\t37151\tSeagrove\tNC\tRandolph County\tH1\n27350\t37151\tSophia\tNC\tRandolph County\tH1\n27355\t37151\tStaley\tNC\tRandolph County\tH1\n27260\t37151\tHigh point\tNC\tRandolph County\tH1\n27239\t37151\tDenton\tNC\tRandolph County\tH1\n27233\t37151\tClimax\tNC\tRandolph County\tH1\n27263\t37151\tHigh point\tNC\tRandolph County\tH1\n27208\t37151\tBennett\tNC\tRandolph County\tH1\n27248\t37151\tFranklinville\tNC\tRandolph County\tH1\n27298\t37151\tLiberty\tNC\tRandolph County\tH1\n27283\t37151\tJulian\tNC\tRandolph County\tH1\n27292\t37151\tLexington\tNC\tRandolph County\tH1\n27316\t37151\tRamseur\tNC\tRandolph County\tH1\n27370\t37151\tTrinity\tNC\tRandolph County\tH1\n28338\t37153\tEllerbe\tNC\tRichmond County\tH1\n27306\t37153\tMount gilead\tNC\tRichmond County\tH1\n28330\t37153\tCordova\tNC\tRichmond County\tH1\n28347\t37153\tHoffman\tNC\tRichmond County\tH1\n27229\t37153\tCandor\tNC\tRichmond County\tH1\n28363\t37153\tMarston\tNC\tRichmond County\tH1\n28367\t37153\tNorman\tNC\tRichmond County\tH1\n28351\t37153\tLaurel hill\tNC\tRichmond County\tH1\n28379\t37153\tRockingham\tNC\tRichmond County\tH1\n28380\t37153\tRockingham\tNC\tRichmond County\tH1\n27281\t37153\tJackson springs\tNC\tRichmond County\tH1\n28345\t37153\tHamlet\tNC\tRichmond County\tH1\n28359\t37155\tLumberton\tNC\tRobeson County\tH1\n28371\t37155\tParkton\tNC\tRobeson County\tH1\n28358\t37155\tLumberton\tNC\tRobeson County\tH1\n28372\t37155\tPembroke\tNC\tRobeson County\tH1\n28375\t37155\tProctorville\tNC\tRobeson County\tH1\n28362\t37155\tMarietta\tNC\tRobeson County\tH1\n28352\t37155\tLaurinburg\tNC\tRobeson County\tH1\n28364\t37155\tMaxton\tNC\tRobeson County\tH1\n28383\t37155\tRowland\tNC\tRobeson County\tH1\n28340\t37155\tFairmont\tNC\tRobeson County\tH1\n28360\t37155\tLumberton\tNC\tRobeson County\tH1\n28384\t37155\tSaint pauls\tNC\tRobeson County\tH1\n28369\t37155\tOrrum\tNC\tRobeson County\tH1\n28377\t37155\tRed springs\tNC\tRobeson County\tH1\n28386\t37155\tShannon\tNC\tRobeson County\tH1\n28378\t37155\tRex\tNC\tRobeson County\tH1\n28357\t37155\tLumber bridge\tNC\tRobeson County\tH1\n27048\t37157\tStoneville\tNC\tRockingham County\tH1\n27326\t37157\tRuffin\tNC\tRockingham County\t
